vi "Get Mapping By Type.vi"(10 "Type":T1, 11 "Mappings":T2[](array[typedef])) -> (3 "index":i32)   [LabVIEW 2013, in "Engine Runtime Interface.lvclass"]
uses:
  Engine Runtime Interface.lvclass
  Engine Configuration/Mappings.ctl
  <vilib>/NI/Tag Bus/tag/Data Type.ctl
  <vilib>/NI/Tag Bus/tag/tag descriptor.lvclass
  Engine Configuration/engine configuration.lvclass
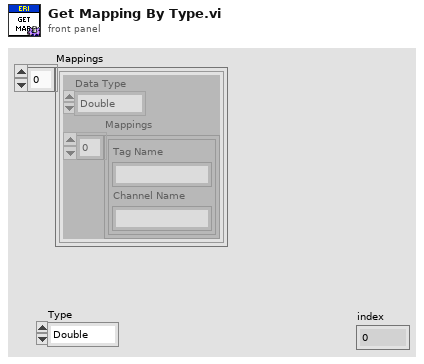
[diagram p1: front panel]
types:
  T1 = typedef "tag bus.lvlib/tag descriptor.lvclass/Data Type.ctl" = enum16{"Double", "Single", "I64", "I32", "I16", "I8", "U64", "U32", "U16", "U8", "Boolean", "String", "Array of Double", "Array of Single", "Array of I64", "Array of I32", "Array of I16", "Array of I8", "Array of U64", "Array of U32", "Array of U16", "Array of U8", "Array of Boolean", "Array of String"}
  T2 = typedef "engine configuration.lvclass/Mappings.ctl" = cluster{"Data Type":T1, "Mappings":cluster{"Tag Name":string, "Channel Name":string}[]}
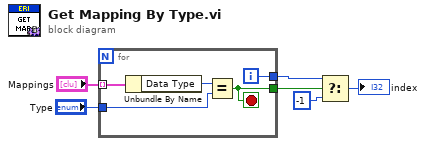
[diagram p0: block diagram]
diagram:
  n1 = for {
    tunnel: "Mappings" -> [w9] mode=indexing
    tunnel: "Type" -> [w10]
    tunnel: [w8] -> w3
    tunnel: [w7] -> w2
    i -> [w8]
    stop <- w7 stop-if-true
    n2 = Unbundle By Name(w9) -> ("Data Type"=w11:T1)
    n3 = Equal?(x=w11, y=w10) -> (x = y?=w7:bool)
  }
  n4 = Select(t=w3, s=w2, f=-1) -> (s? t:f=→"index":i32)
